vi "pixelPitch.vi"(10 "Lens":dbl, 11 "Mag":dbl) -> (3 "PixelPitch":dbl)   [LabVIEW 2011]
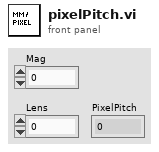
[diagram p1: front panel]
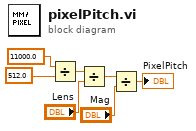
[diagram p0: block diagram]
diagram:
  n1 = Divide(x=11000.0, y=512.0) -> (x/y=w6:dbl)
  n2 = Divide(x=w6, y="Lens") -> (x/y=w7:dbl)
  n3 = Divide(x=w7, y="Mag") -> (x/y=→"PixelPitch":dbl)
